vi "readAndWriteSerial_3102.vi"(8 "error in (no error)":errorcluster {"code" format="%.0x"}, 10 "Write Buffer (\"\")":string="IDN?", 11 "instrument handle":refnum<k15>) -> (0 "error out":errorcluster {"code" format="%.0x"}, 1 "converted number":i32, 2 "Read Buffer":string, 3 "instrument handle out":refnum<k15>)   [LabVIEW 2015, in "SerialCommunication.lvlib"]
uses:
  SerialCommunication.lvlib
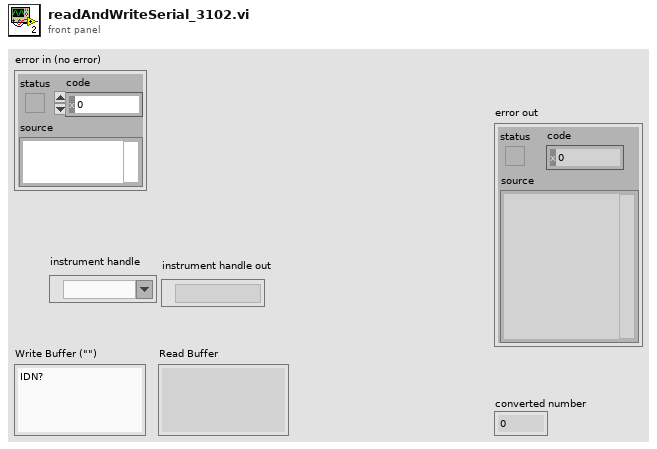
[diagram p1: front panel]
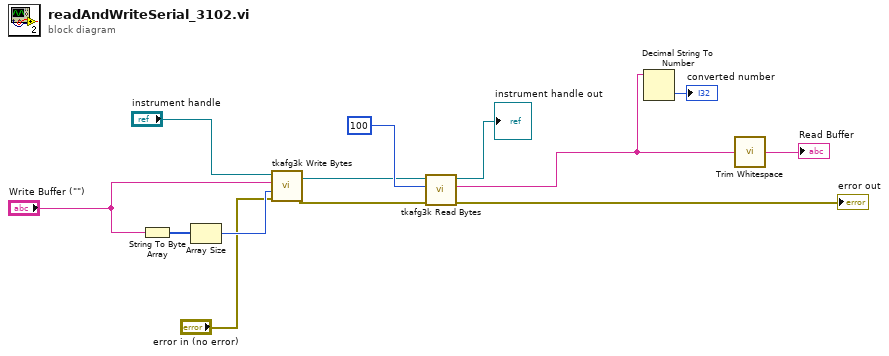
[diagram p0: block diagram]
diagram:
  n1 = String To Byte Array(string="Write Buffer (\"\")") -> (unsigned byte array=w11:u8[])
  n2 = Array Size(array=w11) -> (size(s)=w10:i32)
  n3 = call <instrlib>:"tkafg3k Write Bytes.vi"("error in (no error)"="error in (no error)", "Number of Bytes to Write"=w10, "Write Buffer (\"\")"="Write Buffer (\"\")", "instrument handle"="instrument handle") -> ("error out"=w13:errorcluster, "instrument handle out"=w2:refnum<k15>)  [unwired: 5 in, 1 out]
  n4 = call <instrlib>:"tkafg3k Read Bytes.vi"("error in (no error)"=w13, "Number of Bytes to Read"=i64 100, "instrument handle"=w2) -> ("error out"=→"error out":errorcluster, "Read Buffer"=w4:string, "instrument handle out"=→"instrument handle out":refnum<k15>)  [unwired: 5 in, 1 out]
  n5 = Decimal String To Number(string=w4) -> (number=→"converted number":i32)  [unwired: 2 in, 1 out]
  n6 = call <vilib>:"Trim Whitespace.vi"("string"=w4) -> ("trimmed string"=→"Read Buffer":string)  [unwired: 1 in]
